vi "lead-lag_ctrl.vi"(6 "Mode":T1, 8 "Sampling Time":dbl, 9 "tau":dbl, 10 "alpha":dbl, 11 "Input":dbl) -> (0 "Sampling\nTime Out":dbl, 3 "Output":dbl)   [LabVIEW 2018, in "DiscreteControllers.lvlib"]
doc: "Lead/Lag controller \nImplements (alpha*tau*s+1)/(tau*s+1) in discrete form.\nalpha > 1 (lead), alpha < 1 (lag)\nSelect the appropriate discretization mode."
uses:
  DiscreteControllers.lvlib
  TF_diff_mode.ctl
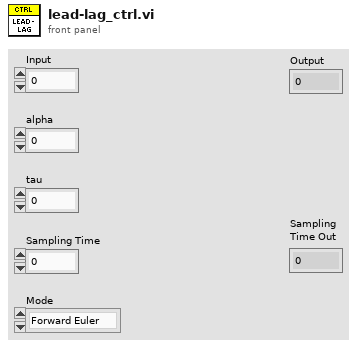
[diagram p1: front panel]
types:
  T1 = typedef "DiscreteControllers.lvlib/TF_diff_mode.ctl" = enum16{"Forward Euler", "Backward Euler", "Tustin (Bilinear)"}
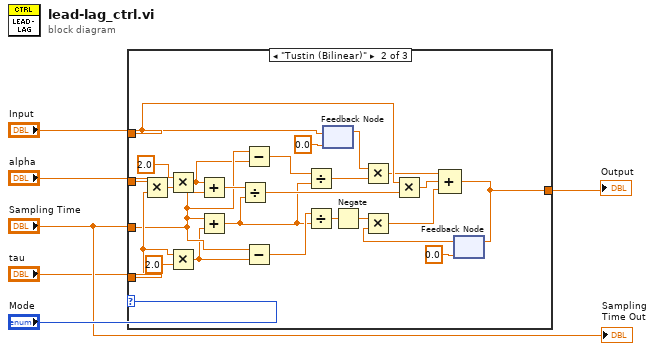
[diagram p0: block diagram]
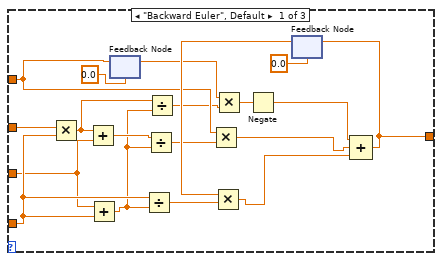
[diagram p2: hidden frame]
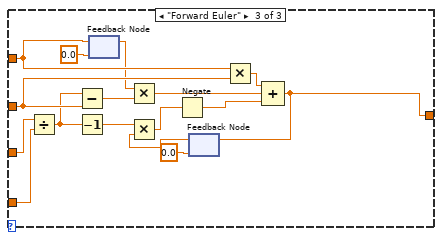
[diagram p3: hidden frame]
diagram:
  n1 = case shown="\"Tustin (Bilinear)\"" "Mode" {
    tunnel: "Input" -> [w17 w42 w64]
    tunnel: "alpha" -> [w23 w50 w62]
    tunnel: "Sampling Time" -> [w7 w38 w66]
    tunnel: "tau" -> [w22 w49 w65]
    tunnel: [w8 w32 w55] -> w1
    frame "Backward Euler", Default {
      n2 = Multiply(x=w23, y=w22) -> (x*y=w16:dbl)
      n3 = Add(x=w16, y=w7) -> (x+y=w19:dbl)
      n4 = Add(x=w7, y=w22) -> (x+y=w15:dbl)
      n5 = feedback #1(0.0 ("Input")) -> (w13:dbl)
      n6 = feedback-in #1(w17) -> ()
      n7 = Divide(x=w22, y=w15) -> (x/y=w21:dbl)
      n8 = Divide(x=w19, y=w15) -> (x/y=w18:dbl)
      n9 = Divide(x=w16, y=w15) -> (x/y=w14:dbl)
      n10 = Multiply(x=w17, y=w18) -> (x*y=w10:dbl)
      n11 = Multiply(x=w13, y=w14) -> (x*y=w12:dbl)
      n12 = Negate(x=w12) -> (-x=w11:dbl)
      n13 = feedback #2(0.0) -> (w20:dbl)
      n14 = Multiply(x=w20, y=w21) -> (x*y=w9:dbl)
      n15 = Compound Arithmetic op=ADD(w11, w10, w9) -> (w8:dbl)
      n16 = feedback-in #2(w8) -> ()
    }
    frame "Tustin (Bilinear)" {
      n17 = Multiply(x=w50, y=w49) -> (x*y=w44:dbl)
      n18 = Multiply(x=2.0, y=w44) -> (x*y=w29:dbl)
      n19 = Multiply(x=w49, y=2.0) -> (x*y=w37:dbl)
      n20 = Add(x=w29, y=w38) -> (x+y=w47:dbl)
      n21 = Add(x=w38, y=w37) -> (x+y=w35:dbl)
      n22 = Divide(x=w47, y=w35) -> (x/y=w46:dbl)
      n23 = Subtract(x=w38, y=w29) -> (x-y=w45:dbl)
      n24 = Subtract(x=w38, y=w37) -> (x-y=w36:dbl)
      n25 = Divide(x=w45, y=w35) -> (x/y=w40:dbl)
      n26 = Divide(x=w36, y=w35) -> (x/y=w28:dbl)
      n27 = feedback-in #3(w42) -> ()
      n28 = feedback #3(0.0 ("Input")) -> (w39:dbl)
      n29 = Negate(x=w28) -> (-x=w27:dbl)
      n30 = Multiply(x=w39, y=w40) -> (x*y=w34:dbl)
      n31 = Multiply(x=w42, y=w46) -> (x*y=w33:dbl)
      n32 = feedback #4(0.0) -> (w30:dbl)
      n33 = Multiply(x=w27, y=w30) -> (x*y=w26:dbl)
      n34 = Compound Arithmetic op=ADD(w34, w33, w26) -> (w32:dbl)
      n35 = feedback-in #4(w32) -> ()
    }
    frame "Forward Euler" {
      n36 = Divide(x=w66, y=w65) -> (x/y=w59:dbl)
      n37 = Subtract(x=w59, y=w62) -> (x-y=w61:dbl)
      n38 = Decrement(x=w59) -> (x-1=w58:dbl)
      n39 = feedback-in #5(w64) -> ()
      n40 = feedback #5(0.0 ("Input")) -> (w60:dbl)
      n41 = Multiply(x=w60, y=w61) -> (x*y=w53:dbl)
      n42 = feedback #6(0.0) -> (w57:dbl)
      n43 = Multiply(x=w58, y=w57) -> (x*y=w56:dbl)
      n44 = Negate(x=w56) -> (-x=w52:dbl)
      n45 = Multiply(x=w64, y=w62) -> (x*y=w51:dbl)
      n46 = Compound Arithmetic op=ADD(w51, w53, w52) -> (w55:dbl)
      n47 = feedback-in #6(w55) -> ()
    }
  }
  "Output" <- w1
  "Sampling\nTime Out" <- "Sampling Time"
